vi "setup_clip_planes.vi"(9 "Graph Range Min/Max":T1, 10 "Axes Properties":T3, 11 "Scene.Object In":refnum<vi>) -> (3 "Scene.Object Out":refnum<vi>)   [LabVIEW 2020, in "3DPC_SurfacePlot.xctl"]
uses:
  <vilib>/Native 3D Graph/xcontrol/3DPC_SurfacePlot.xctl
  <vilib>/Native 3D Graph/typedefs/prop_axes_all.ctl
  <vilib>/Native 3D Graph/typedefs/prop_axes_grid.ctl
  <vilib>/Native 3D Graph/typedefs/prop_axes_ticks.ctl
  <vilib>/Native 3D Graph/typedefs/range_cluster.ctl
  <vilib>/Native 3D Graph/typedefs/min_max.ctl
  <vilib>/Native 3D Graph/typedefs/prop_axes_captions.ctl
  <vilib>/Native 3D Graph/typedefs/prop_axes_labels.ctl
  <vilib>/Native 3D Graph/typedefs/prop_axes_autorange.ctl
  <vilib>/picture/3D Picture Control/NI_3D Picture Control.lvlib
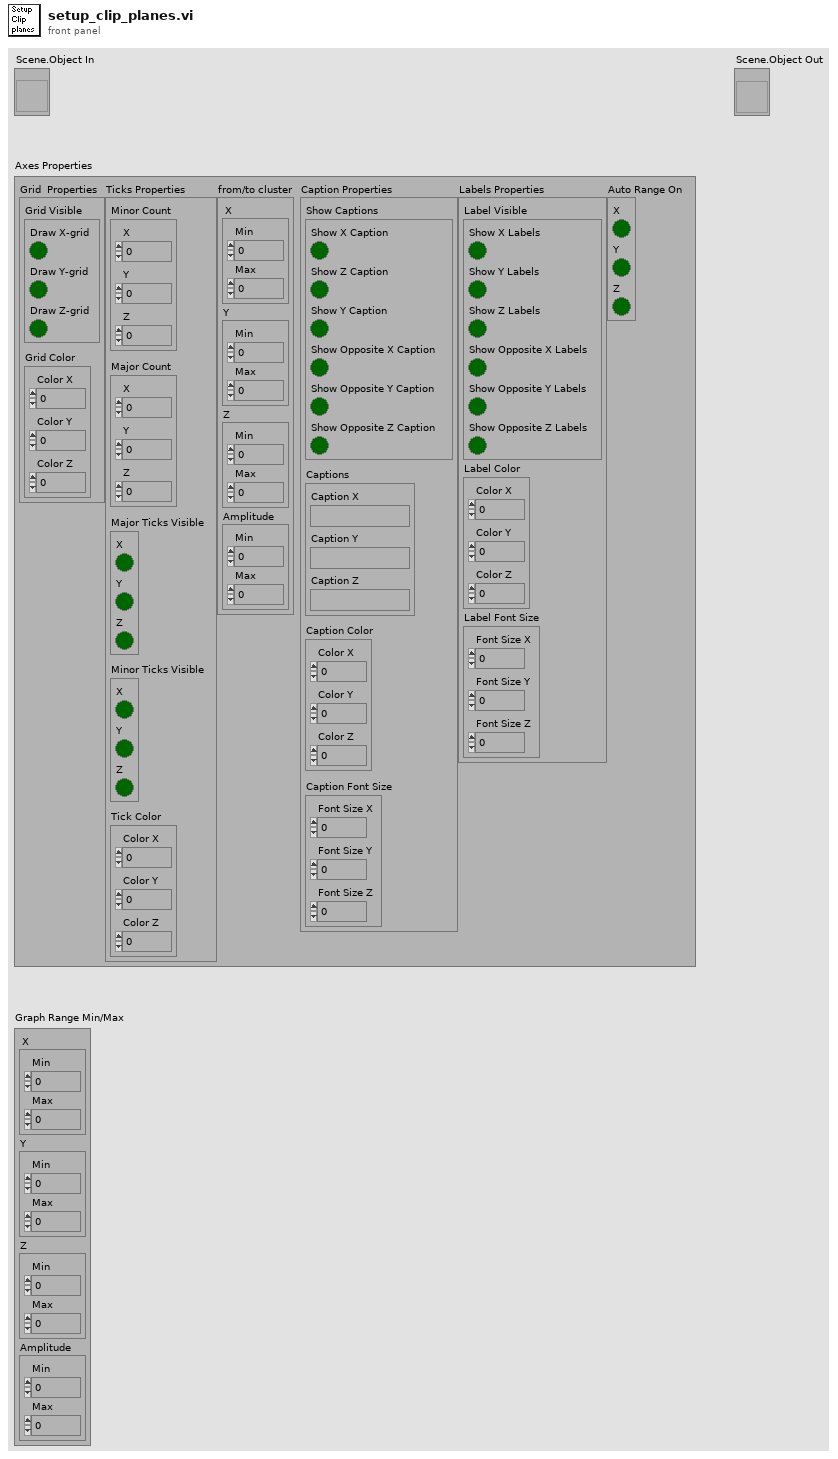
[diagram p1: front panel]
types:
  T1 = typedef "3DPC_SurfacePlot.xctl/range_cluster.ctl" = cluster{"X":T2, "Y":T2, "Z":T2, "Amplitude":T2}
  T2 = typedef "3DPC_SurfacePlot.xctl/min_max.ctl" = cluster{"Min":sgl, "Max":sgl}
  T3 = typedef "3DPC_SurfacePlot.xctl/prop_axes_all.ctl" = cluster{"Grid  Properties":T4, "Ticks Properties":T5, "from/to cluster":T1, "Caption Properties":T6, "Labels Properties":T7, "Auto Range On":T8}
  T4 = typedef "3DPC_SurfacePlot.xctl/prop_axes_grid.ctl" = cluster{"Grid Visible":cluster{"Draw X-grid":bool, "Draw Y-grid":bool, "Draw Z-grid":bool}, "Grid Color":cluster{"Color X":u32, "Color Y":u32, "Color Z":u32}}
  T5 = typedef "3DPC_SurfacePlot.xctl/prop_axes_ticks.ctl" = cluster{"Minor Count":cluster{"X":i32, "Y":i32, "Z":i32}, "Major Count":cluster{"X":i32, "Y":i32, "Z":i32}, "Major Ticks Visible":cluster{"X":bool, "Y":bool, "Z":bool}, "Minor Ticks Visible":cluster{"X":bool, "Y":bool, "Z":bool}, "Tick Color":cluster{"Color X":u32, "Color Y":u32, "Color Z":u32}}
  T6 = typedef "3DPC_SurfacePlot.xctl/prop_axes_captions.ctl" = cluster{"Show Captions":cluster{"Show X Caption":bool, "Show Z Caption":bool, "Show Y Caption":bool, "Show Opposite X Caption":bool, "Show Opposite Y Caption":bool, "Show Opposite Z Caption":bool}, "Captions":cluster{"Caption X":string, "Caption Y":string, "Caption Z":string}, "Caption Color":cluster{"Color X":u32, "Color Y":u32, "Color Z":u32}, "Caption Font Size":cluster{"Font Size X":i16, "Font Size Y":i16, "Font Size Z":i16}}
  T7 = typedef "3DPC_SurfacePlot.xctl/prop_axes_labels.ctl" = cluster{"Label Visible":cluster{"Show X Labels":bool, "Show Y Labels":bool, "Show Z Labels":bool, "Show Opposite X Labels":bool, "Show Opposite Y Labels":bool, "Show Opposite Z Labels":bool}, "Label Color":cluster{"Color X":u32, "Color Y":u32, "Color Z":u32}, "Label Font Size":cluster{"Font Size X":i16, "Font Size Y":i16, "Font Size Z":i16}}
  T8 = typedef "3DPC_SurfacePlot.xctl/prop_axes_autorange.ctl" = cluster{"X":bool, "Y":bool, "Z":bool}
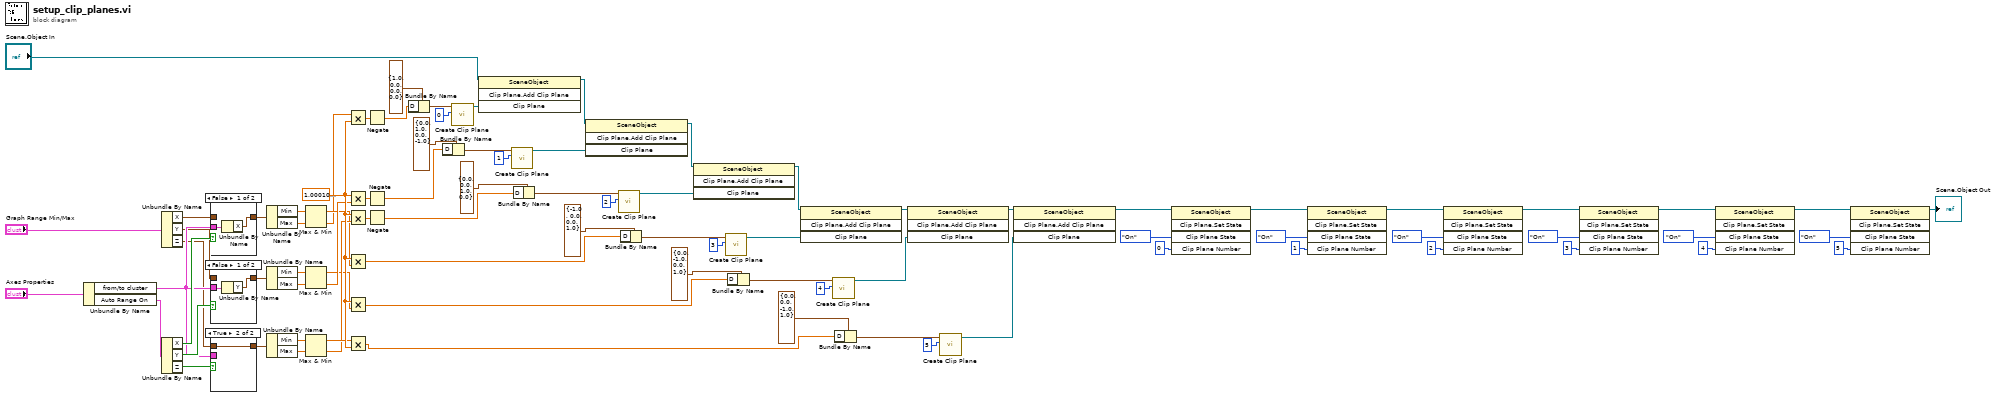
[diagram p0: block diagram]
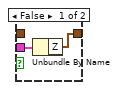
[diagram p2: hidden frame]
diagram:
  w14 = sgl 1.0001 ("y")
  n1 = Unbundle By Name("Axes Properties") -> ("from/to cluster"=w42:T1, "Auto Range On"=w46:T8)
  n2 = Unbundle By Name("Graph Range Min/Max") -> ("X"=w41:T2, "Y"=w40:T2, "Z"=w39:T2)
  n3 = Unbundle By Name(w46) -> ("X"=w45:bool, "Y"=w44:bool, "Z"=w43:bool)
  n4 = case shown="False" w45 {
    tunnel: w42 -> [w86 _]
    tunnel: [w85 w87] -> w31
    tunnel: w41 -> [_ w87]
    frame False {
      n5 = Unbundle By Name(w86) -> ("X"=w85:T2)
    }
    frame True {
    }
  }
  n6 = case shown="False" w44 {
    tunnel: w42 -> [w89 _]
    tunnel: [w88 w90] -> w32
    tunnel: w40 -> [_ w90]
    frame False {
      n7 = Unbundle By Name(w89) -> ("Y"=w88:T2)
    }
    frame True {
    }
  }
  n8 = case shown="True" w43 {
    tunnel: w42 -> [w92 _]
    tunnel: [w91 w93] -> w38
    tunnel: w39 -> [_ w93]
    frame False {
      n9 = Unbundle By Name(w92) -> ("Z"=w91:T2)
    }
    frame True {
    }
  }
  n10 = Unbundle By Name(w31) -> ("Min"=w2:sgl, "Max"=w4:sgl)
  n11 = Unbundle By Name(w32) -> ("Min"=w8:sgl, "Max"=w6:sgl)
  n12 = Unbundle By Name(w38) -> ("Min"=w12:sgl, "Max"=w11:sgl)
  n13 = Max & Min(x=w2, y=w4) -> (max(x,y)=w3:sgl, min(x,y)=w1:sgl)
  n14 = Max & Min(x=w8, y=w6) -> (max(x,y)=w5:sgl, min(x,y)=w7:sgl)
  n15 = Max & Min(x=w12, y=w11) -> (max(x,y)=w10:sgl, min(x,y)=w9:sgl)
  n16 = Multiply(x=w1, y=w14) -> (x*y=w17:sgl)
  n17 = Multiply(x=w14, y=w7) -> (x*y=w16:sgl)
  n18 = Multiply(x=w14, y=w9) -> (x*y=w19:sgl)
  n19 = Multiply(x=w14, y=w3) -> (x*y=w15:sgl)
  n20 = Multiply(x=w14, y=w5) -> (x*y=w13:sgl)
  n21 = Multiply(x=w10, y=w14) -> (x*y=w18:sgl)
  n22 = Negate(x=w17) -> (-x=w20:sgl)
  n23 = Negate(x=w16) -> (-x=w21:sgl)
  n24 = Negate(x=w19) -> (-x=w22:sgl)
  n25 = Bundle By Name(cluster=cluster{"A":sgl, "B":sgl, "C":sgl, "D":sgl} {"A"=1.0, "B"=0.0, "C"=0.0, "D"=0.0} ("Plane"), "D"=w20) -> (w23:cluster{"A":sgl, "B":sgl, "C":sgl, "D":sgl})
  n26 = Bundle By Name(cluster=cluster{"A":sgl, "B":sgl, "C":sgl, "D":sgl} {"A"=0.0, "B"=1.0, "C"=0.0, "D"=-1.0} ("Plane"), "D"=w21) -> (w25:cluster{"A":sgl, "B":sgl, "C":sgl, "D":sgl})
  n27 = call <vilib>:"Create Clip Plane.vi"("Number"=0, "Plane"=w23) -> ("New Clip Plane Refnum"=w83:refnum<vi>)  [unwired: 1 in, 8 out]
  n28 = invoke class="SceneObject" method="Clip Plane.Add Clip Plane"(reference="Scene.Object In", "Clip Plane"=w83) -> (reference out=w82:refnum<vi>)  [unwired: 2 in, 3 out]
  n29 = call <vilib>:"Create Clip Plane.vi"("Number"=1, "Plane"=w25) -> ("New Clip Plane Refnum"=w81:refnum<vi>)  [unwired: 1 in, 8 out]
  n30 = Bundle By Name(cluster=cluster{"A":sgl, "B":sgl, "C":sgl, "D":sgl} {"A"=0.0, "B"=0.0, "C"=1.0, "D"=0.0} ("Plane"), "D"=w22) -> (w27:cluster{"A":sgl, "B":sgl, "C":sgl, "D":sgl})
  n31 = invoke class="SceneObject" method="Clip Plane.Add Clip Plane"(reference=w82, "Clip Plane"=w81) -> (reference out=w80:refnum<vi>)  [unwired: 2 in, 3 out]
  n32 = call <vilib>:"Create Clip Plane.vi"("Number"=2, "Plane"=w27) -> ("New Clip Plane Refnum"=w79:refnum<vi>)  [unwired: 1 in, 8 out]
  n33 = Bundle By Name(cluster=cluster{"A":sgl, "B":sgl, "C":sgl, "D":sgl} {"A"=-1.0, "B"=0.0, "C"=0.0, "D"=1.0} ("Plane"), "D"=w15) -> (w28:cluster{"A":sgl, "B":sgl, "C":sgl, "D":sgl})
  n34 = invoke class="SceneObject" method="Clip Plane.Add Clip Plane"(reference=w80, "Clip Plane"=w79) -> (reference out=w70:refnum<vi>)  [unwired: 2 in, 3 out]
  n35 = call <vilib>:"Create Clip Plane.vi"("Number"=3, "Plane"=w28) -> ("New Clip Plane Refnum"=w71:refnum<vi>)  [unwired: 1 in, 8 out]
  n36 = Bundle By Name(cluster=cluster{"A":sgl, "B":sgl, "C":sgl, "D":sgl} {"A"=0.0, "B"=-1.0, "C"=0.0, "D"=1.0} ("Plane"), "D"=w13) -> (w34:cluster{"A":sgl, "B":sgl, "C":sgl, "D":sgl})
  n37 = invoke class="SceneObject" method="Clip Plane.Add Clip Plane"(reference=w70, "Clip Plane"=w71) -> (reference out=w68:refnum<vi>)  [unwired: 2 in, 3 out]
  n38 = call <vilib>:"Create Clip Plane.vi"("Number"=4, "Plane"=w34) -> ("New Clip Plane Refnum"=w72:refnum<vi>)  [unwired: 1 in, 8 out]
  n39 = Bundle By Name(cluster=cluster{"A":sgl, "B":sgl, "C":sgl, "D":sgl} {"A"=0.0, "B"=0.0, "C"=-1.0, "D"=1.0} ("Plane"), "D"=w18) -> (w36:cluster{"A":sgl, "B":sgl, "C":sgl, "D":sgl})
  n40 = invoke class="SceneObject" method="Clip Plane.Add Clip Plane"(reference=w68, "Clip Plane"=w72) -> (reference out=w69:refnum<vi>)  [unwired: 2 in, 3 out]
  n41 = call <vilib>:"Create Clip Plane.vi"("Number"=5, "Plane"=w36) -> ("New Clip Plane Refnum"=w73:refnum<vi>)  [unwired: 1 in, 8 out]
  n42 = invoke class="SceneObject" method="Clip Plane.Add Clip Plane"(reference=w69, "Clip Plane"=w73) -> (reference out=w57:refnum<vi>)  [unwired: 2 in, 3 out]
  n43 = invoke class="SceneObject" method="Clip Plane.Set State"(reference=w57, "Clip Plane State"=enum16{"Inherit Value", "Off", "On"}."On", "Clip Plane Number"=0) -> (reference out=w54:refnum<vi>)  [unwired: 2 in, 4 out]
  n44 = invoke class="SceneObject" method="Clip Plane.Set State"(reference=w54, "Clip Plane State"=enum16{"Inherit Value", "Off", "On"}."On", "Clip Plane Number"=1) -> (reference out=w53:refnum<vi>)  [unwired: 2 in, 4 out]
  n45 = invoke class="SceneObject" method="Clip Plane.Set State"(reference=w53, "Clip Plane State"=enum16{"Inherit Value", "Off", "On"}."On", "Clip Plane Number"=2) -> (reference out=w52:refnum<vi>)  [unwired: 2 in, 4 out]
  n46 = invoke class="SceneObject" method="Clip Plane.Set State"(reference=w52, "Clip Plane State"=enum16{"Inherit Value", "Off", "On"}."On", "Clip Plane Number"=3) -> (reference out=w51:refnum<vi>)  [unwired: 2 in, 4 out]
  n47 = invoke class="SceneObject" method="Clip Plane.Set State"(reference=w51, "Clip Plane State"=enum16{"Inherit Value", "Off", "On"}."On", "Clip Plane Number"=4) -> (reference out=w50:refnum<vi>)  [unwired: 2 in, 4 out]
  n48 = invoke class="SceneObject" method="Clip Plane.Set State"(reference=w50, "Clip Plane State"=enum16{"Inherit Value", "Off", "On"}."On", "Clip Plane Number"=5) -> (reference out=→"Scene.Object Out":refnum<vi>)  [unwired: 2 in, 4 out]
